vi "pressure caliberation - v2.vi"() -> ()   [LabVIEW 2018]
uses:
  <vilib>/ptbypt/NI_PtbyPt.lvlib
panel:
  out "M7 5":dbl
  out "M7 4":dbl
  out "M2 3":dbl
  out "M4 2":dbl
  out "M1":dbl
  out "M-8":dbl(graph)
  out "M-1":dbl(graph)
  out "M-12":dbl(graph)
  out "M-11":dbl(graph)
  out "M-6":dbl(graph)
  out "M-7":dbl(graph)
  out "M-2":dbl(graph)
  out "M-4":dbl(graph)
  in  "stop (F) 3":bool caption="stop (F)"
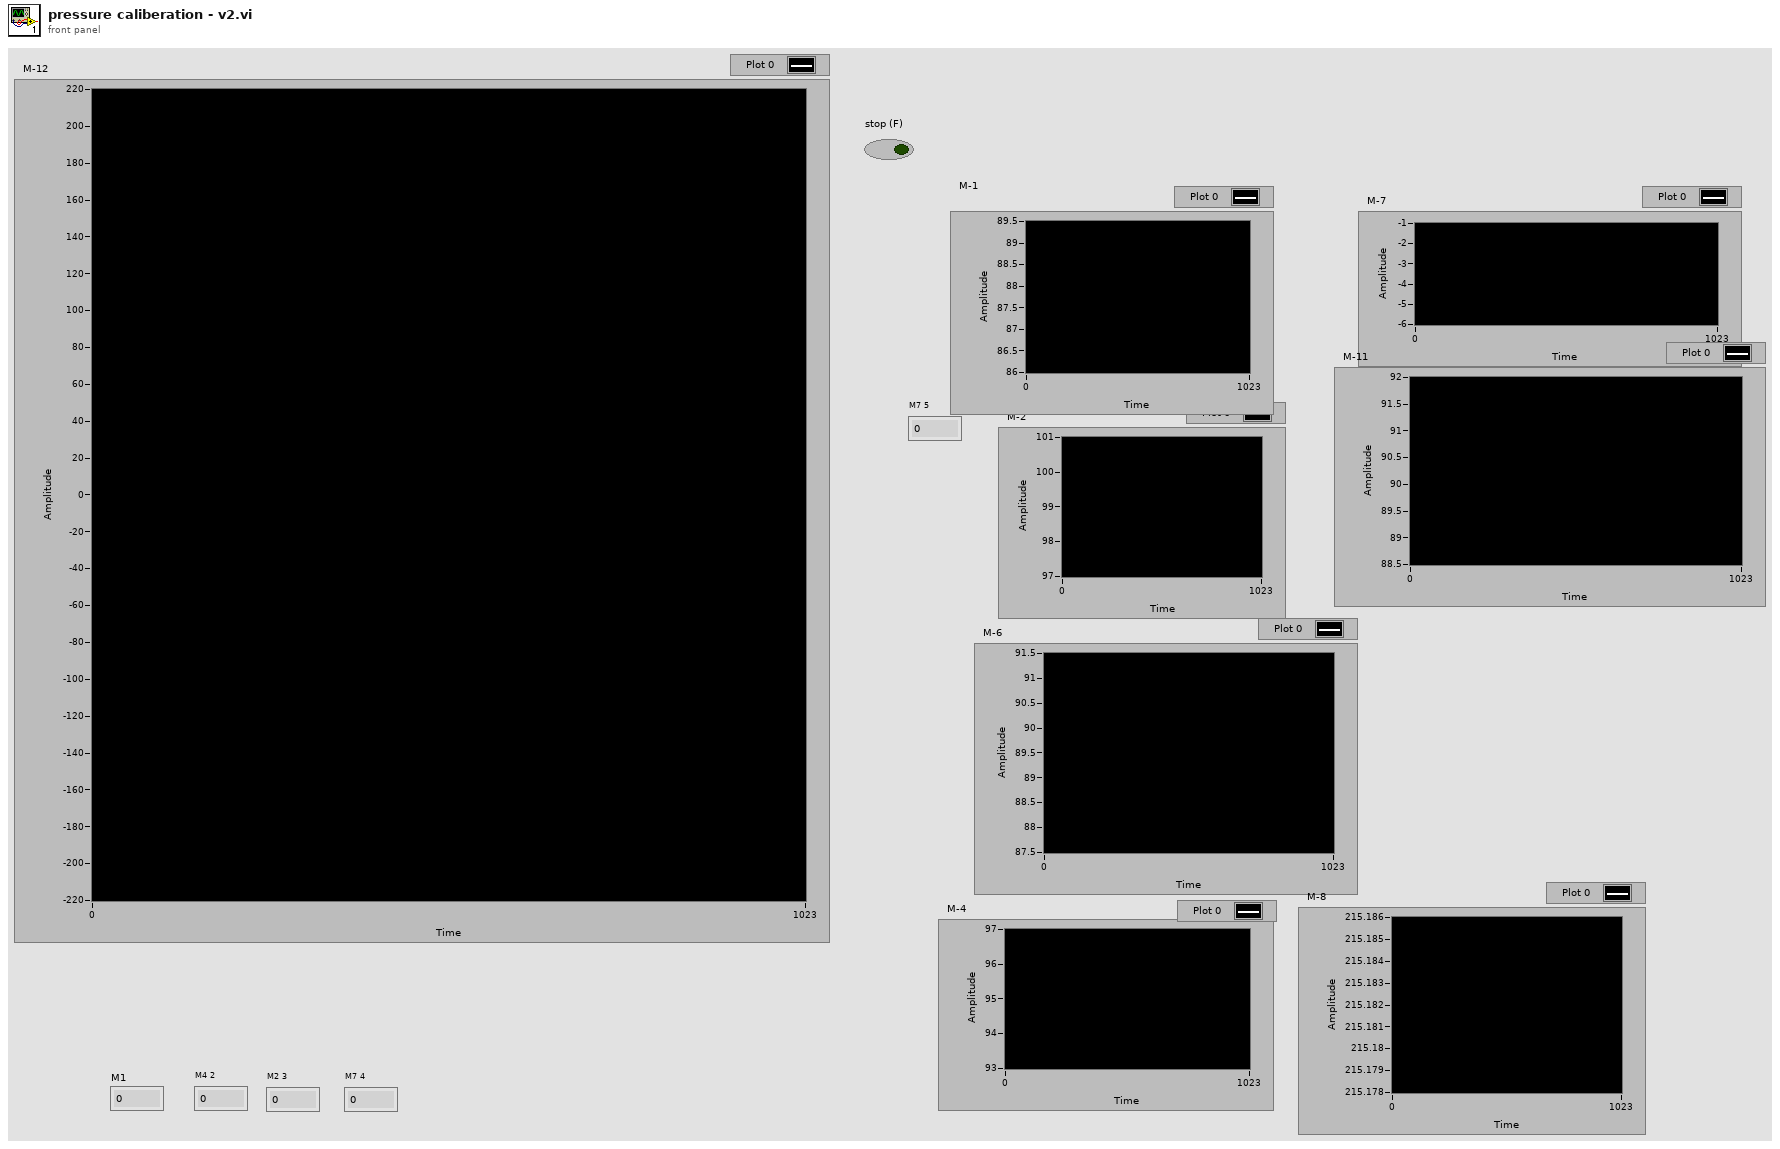
[diagram p1: front panel]
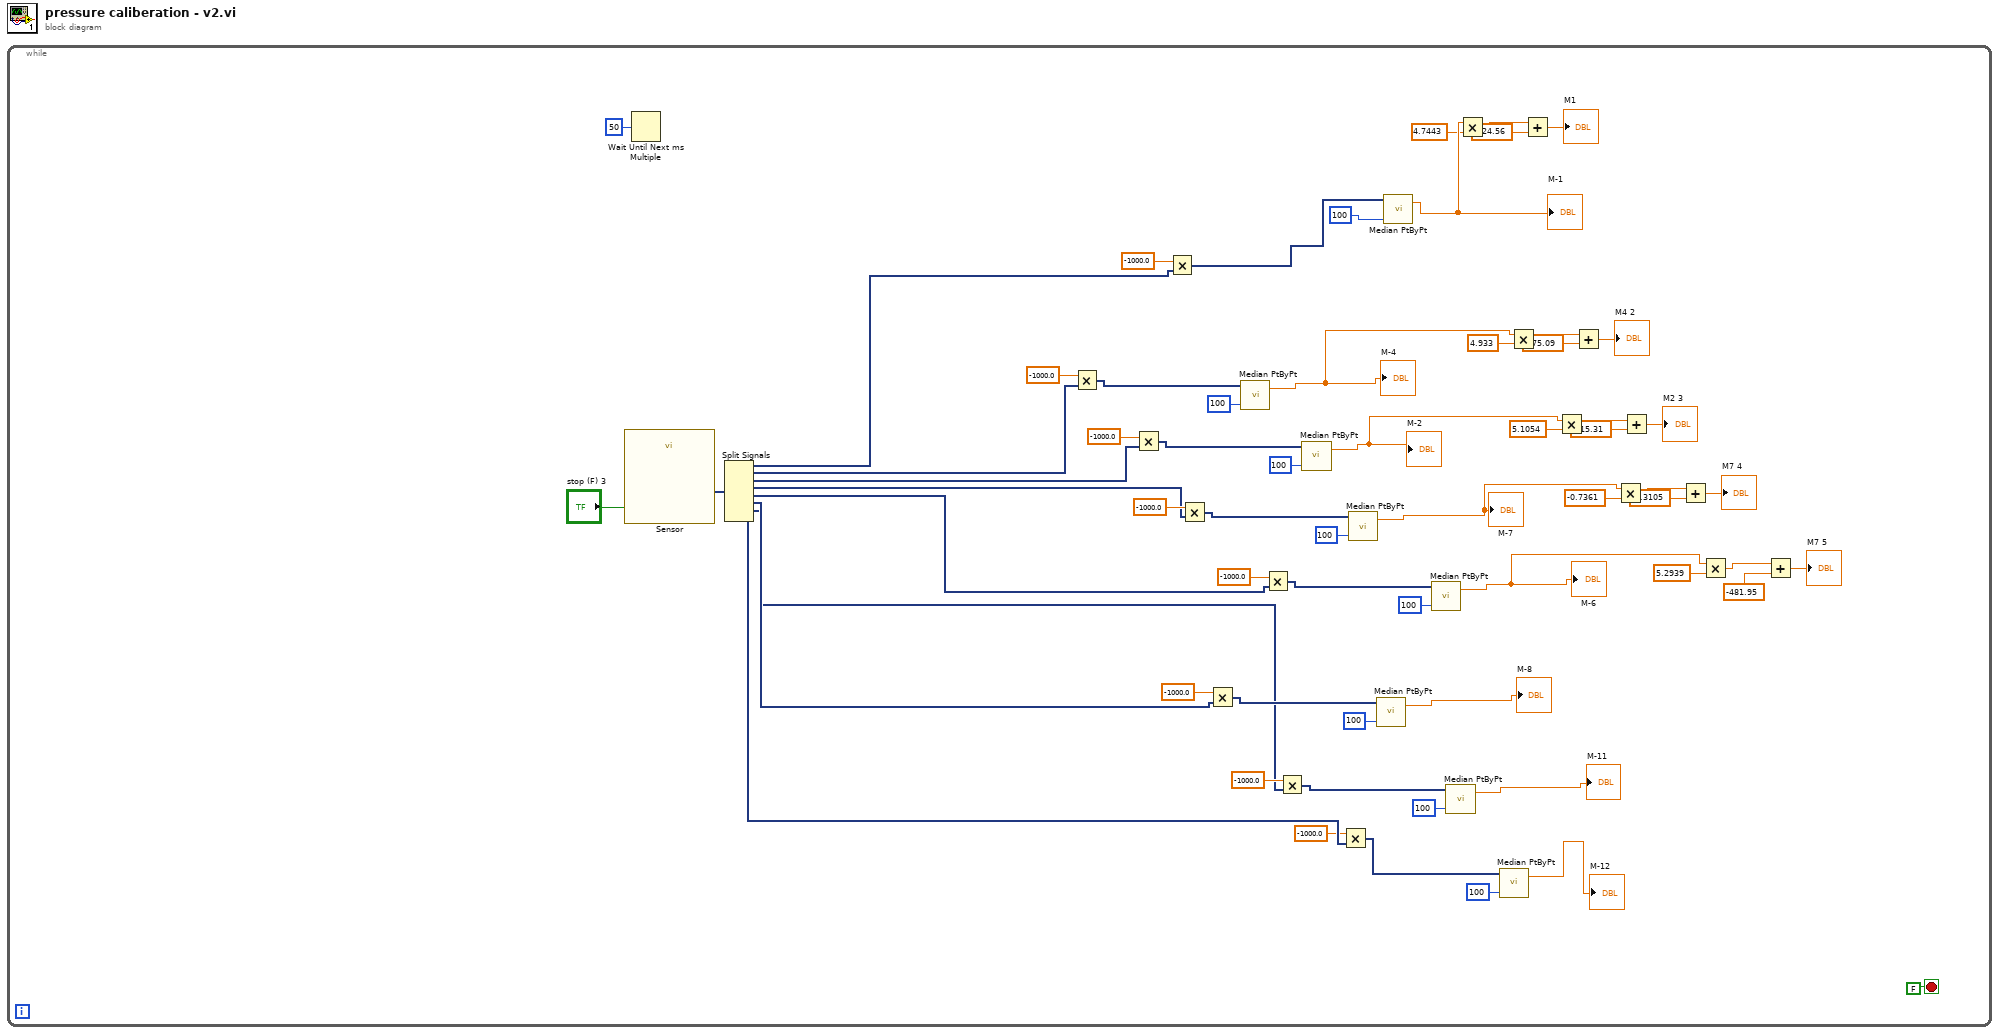
[diagram p0: block diagram]
diagram:
  n1 = while {
    stop <- FALSE stop-if-true
    n2 = call "Sensor"("stop (T)"="stop (F) 3") -> ("data"=w21:dynamicdata)  [unwired: 16 in, 2 out]
    n3 = Wait Until Next ms Multiple(millisecond multiple=u32 50) -> ()  [unwired: 1 out]
    n4 = Split Signals(w21) -> (w1:dynamicdata, w20:dynamicdata, w19:dynamicdata, w18:dynamicdata, w17:dynamicdata, w16:dynamicdata, w15:dynamicdata, w11:dynamicdata)  [unwired: 8 in]
    n5 = Multiply(x=-1000.0, y=w20) -> (x*y=w61:dynamicdata)
    n6 = Multiply(x=-1000.0, y=w19) -> (x*y=w58:dynamicdata)
    n7 = Multiply(x=-1000.0, y=w1) -> (x*y=w9:dynamicdata)
    n8 = Multiply(x=-1000.0, y=w18) -> (x*y=w55:dynamicdata)
    n9 = Multiply(x=-1000.0, y=w16) -> (x*y=w45:dynamicdata)
    n10 = call <vilib>:"Median PtByPt.vi"("sample length"=100, "x"=w61) -> ("median"=w39:dbl)  [unwired: 2 in, 1 out]
    "M-4" <- w39
    n11 = Multiply(x=-1000.0, y=w17) -> (x*y=w52:dynamicdata)
    n12 = Multiply(x=-1000.0, y=w15) -> (x*y=w49:dynamicdata)
    n13 = call <vilib>:"Median PtByPt.vi"("sample length"=100, "x"=w58) -> ("median"=w34:dbl)  [unwired: 2 in, 1 out]
    "M-2" <- w34
    n14 = Multiply(x=-1000.0, y=w11) -> (x*y=w14:dynamicdata)
    n15 = call <vilib>:"Median PtByPt.vi"("sample length"=100, "x"=w55) -> ("median"=w29:dbl)  [unwired: 2 in, 1 out]
    "M-7" <- w29
    n16 = call <vilib>:"Median PtByPt.vi"("sample length"=100, "x"=w45) -> ("median"=→"M-8":dbl)  [unwired: 2 in, 1 out]
    n17 = call <vilib>:"Median PtByPt.vi"("sample length"=100, "x"=w9) -> ("median"=w8:dbl)  [unwired: 2 in, 1 out]
    "M-1" <- w8
    n18 = call <vilib>:"Median PtByPt.vi"("sample length"=100, "x"=w52) -> ("median"=w24:dbl)  [unwired: 2 in, 1 out]
    "M-6" <- w24
    n19 = call <vilib>:"Median PtByPt.vi"("sample length"=100, "x"=w49) -> ("median"=→"M-11":dbl)  [unwired: 2 in, 1 out]
    n20 = Multiply(x=w8, y=4.7443) -> (x*y=w7:dbl)
    n21 = call <vilib>:"Median PtByPt.vi"("sample length"=100, "x"=w14) -> ("median"=→"M-12":dbl)  [unwired: 2 in, 1 out]
    n22 = Multiply(x=w39, y=4.933) -> (x*y=w42:dbl)
    n23 = Add(x=w7, y=-424.56) -> (x+y=→"M1":dbl)
    n24 = Multiply(x=w34, y=5.1054) -> (x*y=w37:dbl)
    n25 = Add(x=w42, y=-475.09) -> (x+y=→"M4 2":dbl)
    n26 = Multiply(x=w29, y=-0.7361) -> (x*y=w32:dbl)
    n27 = Add(x=w37, y=-515.31) -> (x+y=→"M2 3":dbl)
    n28 = Add(x=w32, y=-1.3105) -> (x+y=→"M7 4":dbl)
    n29 = Multiply(x=w24, y=5.2939) -> (x*y=w27:dbl)
    n30 = Add(x=w27, y=-481.95) -> (x+y=→"M7 5":dbl)
  }
